vi "Set Range.vi"(8 "Error In":errorcluster, 10 "Range":T1, 11 "Graph in":refnum<class "Graph.lvclass">) -> (0 "Error Out":errorcluster, 3 "Graph out":refnum<class "Graph.lvclass">)   [LabVIEW 2019, in "Graph.lvclass"]
uses:
  Graph.lvclass
  Public/Controls/Range.ctl
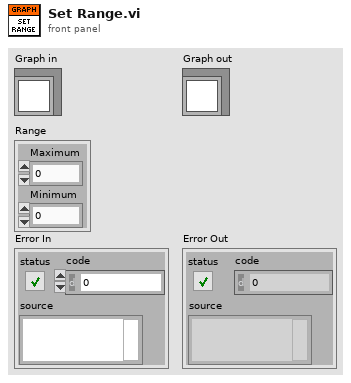
[diagram p1: front panel]
types:
  T1 = typedef "Graph.lvclass/Range.ctl" = cluster{"Maximum":i32, "Minimum":i32}
  T2 = typedef "Graph.lvclass/Data.ctl" = cluster{"Height":u32, "Width":u32, "Range":T1, "Data":i32[], "Fill To":T3}
  T3 = typedef "Graph.lvclass/Fill To.ctl" = enum16{"None", "Zero", "Inf", "-Inf"}
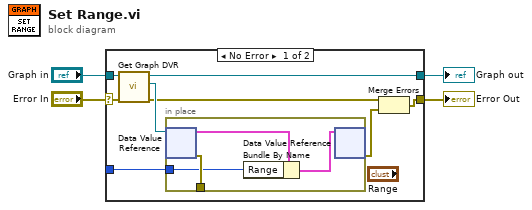
[diagram p0: block diagram]
diagram:
  n1 = case shown="No Error" "Error In" {
    selector: "Error In" -> [w8 w17]
    tunnel: [w11 w17] -> w1
    tunnel: [w6 w18] -> w2
    tunnel: "Graph in" -> [w9 w18]
    tunnel: _ -> [w10 _]
    frame No Error {
      n2 = call "Get Graph DVR.vi"("Error In"=w8, "Graph In"=w9) -> ("Error Out"=w5:errorcluster, "DVR"=w7:refnum<data-value>, "Graph Out"=w6:refnum<class "Graph.lvclass">)  [unwired: 7 in]
      n3 = in-place {
        in-place-border: [w16] -> _
        in-place-border: w10 -> [w13]
        n4 = in-place-dvr #1(w7) -> (w15:T2, w16:errorcluster)
        n5 = Bundle By Name(cluster=w15, "Range"=w13) -> (w14:T2)
        n6 = in-place-dvr #1(w14) -> (w12:errorcluster)  [unwired: 1 out]
      }
      n7 = Merge Errors(w5, w12) -> (w11:errorcluster)
    }
    frame Error {
    }
  }
  "Graph out" <- w2
  "Error Out" <- w1
